vi "user.email.vi"(8 "error in":errorcluster, 11 "User in":refnum<class "User.lvclass">) -> (0 "error out":errorcluster, 2 "user email":string, 3 "User out":refnum<class "User.lvclass">)   [LabVIEW 2020, in "User.lvclass"]
doc: "Returns the user's email."
uses:
  User.lvclass
  User.lvclass/User.ctl
  client.lvlib
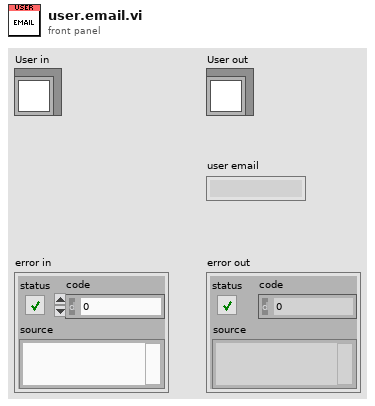
[diagram p1: front panel]
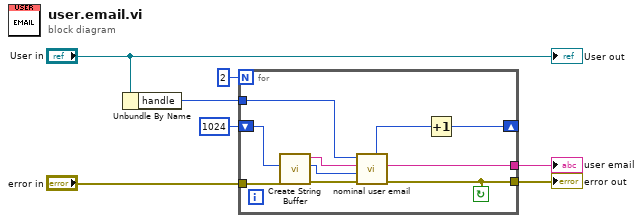
[diagram p0: block diagram]
diagram:
  n1 = Unbundle By Name("User in") -> ("handle"=w3:i32)
  n2 = for {
    N: 2 -> [_]
    tunnel: w3 -> [w17]
    tunnel: [w16] -> w1
    shift-right: [w9] -> _
    shift-left: 1024 ("Buffer Size (1024)") -> [w13]
    tunnel: [w10] -> w2
    tunnel: "error in" -> [w8]
    stop <- w10 continue-if-true
    n3 = call "Create String Buffer.vi"("error in"=w8, "Buffer Size (1024)"=w13) -> ("error out"=w12:errorcluster, "dub Buffer Size"=w14:i32, "String Buffer"=w15:string)  [unwired: 7 in]
    n4 = call "nominal user email.vi"("error in (no error)"=w12, "cap"=w14, "buf"=w15, "user"=w17) -> ("error out"=w10:errorcluster, "buf out"=w16:string, "out_needed out"=w11:u32)  [unwired: 4 in, 1 out]
    n5 = Increment(x=w11) -> (x+1=w9:u32)
  }
  "error out" <- w2
  "user email" <- w1
  "User out" <- "User in"
